vi "Rename State.vi"(0 "Tosca in":refnum<class "Parameters.lvclass">, 5 "stateIndex":i32, 7 "New name":string) -> (4 "Tosca out":refnum<class "Parameters.lvclass">, 8 "accepted":bool)   [LabVIEW 2020, in "Parameters.lvclass"]
uses:
  Parameters.lvclass
  Parameters.lvclass/Parameters.ctl
  State/State.lvclass/State.ctl
  State/Read Name.vi
  State/Write Name.vi
  State/State.lvclass
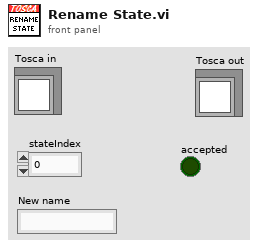
[diagram p1: front panel]
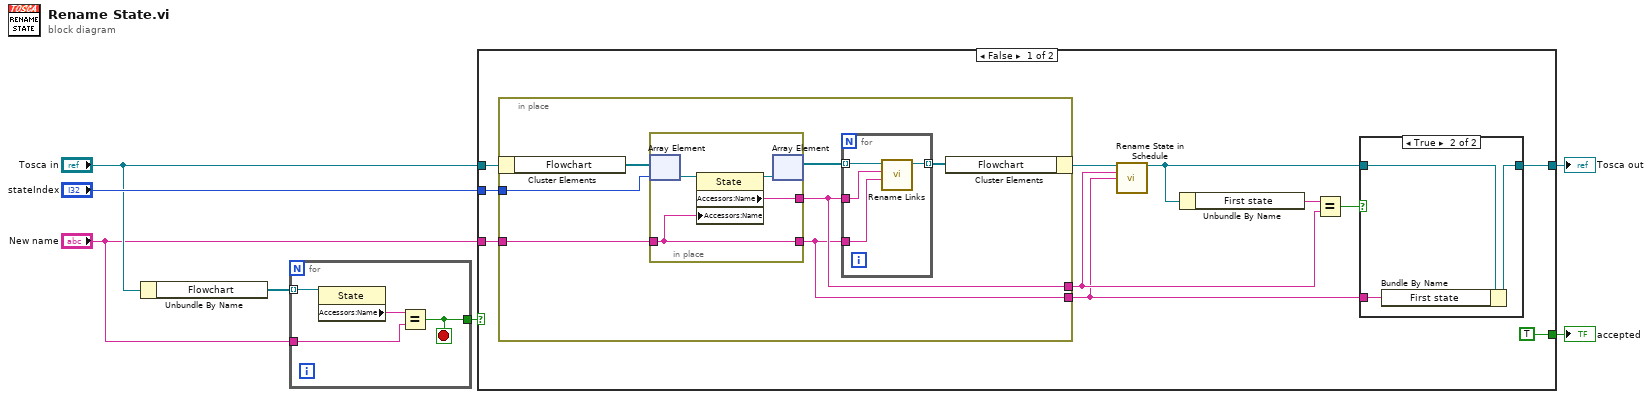
[diagram p0: block diagram]
diagram:
  n1 = Unbundle By Name("Tosca in") -> ("Flowchart"=w4:refnum<class "State.lvclass">[])
  n2 = for {
    tunnel: w4 -> [w11] mode=indexing
    tunnel: "New name" -> [w9]
    tunnel: [w8] -> w2
    stop <- w8 stop-if-true
    n3 = property class="State"(reference=w11) -> ("Accessors:Name"=w10:string)  [unwired: 1 in, 2 out]
    n4 = Equal?(x=w10, y=w9) -> (x = y?=w8:bool)
  }
  n5 = case shown="False" w2 {
    tunnel: [w17 w42] -> w7
    tunnel: "stateIndex" -> [w22 _]
    tunnel: "Tosca in" -> [w21 w42]
    tunnel: "New name" -> [w20 _]
    tunnel: [TRUE _] -> w1
    frame False {
      n6 = in-place {
        in-place-border: w22 -> [w28]
        in-place-border: w20 -> [w27]
        in-place-border: [w24] -> w13
        in-place-border: [w23] -> w12
        n7 = in-place-cluster #1(w21) -> ("Flowchart"=w29:refnum<class "State.lvclass">[])
        n8 = in-place {
          in-place-border: w27 -> [w34]
          in-place-border: [w35] -> w24
          in-place-border: [w34] -> w23
          n9 = in-place-array #2(w29, w28) -> (w37:refnum<class "State.lvclass">)
          n10 = property class="State"(reference=w37, "Accessors:Name"=w34) -> (reference out=w36:refnum<class "State.lvclass">, "Accessors:Name"=w35:string)  [unwired: 1 in, 1 out]
          n11 = in-place-array #2(w36) -> (w26:refnum<class "State.lvclass">[])  [unwired: 1 out]
        }
        n12 = for {
          tunnel: w24 -> [w32]
          tunnel: w26 -> [w33] mode=indexing
          tunnel: [w30] -> w25 mode=indexing
          tunnel: w23 -> [w31]
          n13 = call "Rename Links.vi"("New Name"=w31, "Old Name"=w32, "State in"=w33) -> ("State out"=w30:refnum<class "State.lvclass">)  [unwired: 7 in, 1 out]
        }
        n14 = in-place-cluster #1("Flowchart"=w25) -> (w15:refnum<class "Parameters.lvclass">)
      }
      n15 = call "Rename State in Schedule.vi"("Tosca in"=w15, "Old Name"=w13, "New Name"=w12) -> ("Tosca out"=w14:refnum<class "Parameters.lvclass">)  [unwired: 11 in, 1 out]
      n16 = Unbundle By Name(w14) -> ("First state"=w18:string)
      n17 = Equal?(x=w18, y=w13) -> (x = y?=w16:bool)
      n18 = case shown="True" w16 {
        tunnel: [w38 w40] -> w17
        tunnel: w14 -> [w38 w41]
        tunnel: w12 -> [_ w39]
        frame False {
        }
        frame True {
          n19 = Bundle By Name(cluster=w41, "First state"=w39) -> (w40:refnum<class "Parameters.lvclass">)
        }
      }
    }
    frame True {
      # "Duplicate name"
    }
  }
  "Tosca out" <- w7
  "accepted" <- w1
